vi "Read settings.vi"(8 "error in (no error)":errorcluster, 9 "force loading?":bool=TRUE, 10 "settings name":string, 11 "Autofocus in":refnum<class "Autofocus.lvclass">) -> (0 "error out":errorcluster, 1 "loaded?":bool, 2 "setting name":string, 3 "Autofocus out":refnum<class "Autofocus.lvclass">)   [LabVIEW 2012, in "Autofocus.lvclass"]
uses:
  Autofocus.lvclass
  <vilib>/Distrio/Murmex/Murmex/Murmex.lvclass
  Autofocus.lvclass/Autofocus.ctl
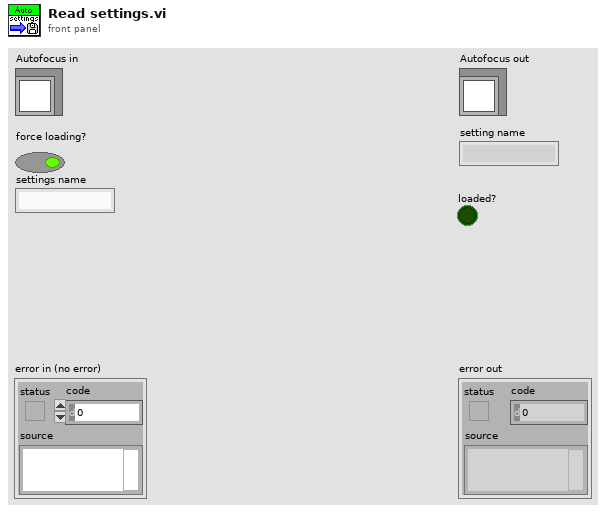
[diagram p1: front panel]
types:
  T1 = typedef "Autofocus.lvclass/settings cluster.ctl" = cluster{"Sharpness measure":T2, "ROI size":T3, "Search Algorithm":T4, "Region sampling":bool, "HC step size":dbl[unit], "current_position_focus":dbl[unit], "threshold":dbl, "brightest percentage":dbl, "number_of_checkpoints":u16, "current_stack_x":dbl[unit], "current_stack_y":dbl[unit], "curent_stack_z1":dbl[unit], "current_stack_z2":dbl[unit], "number_of_stacks":u16, "focus_start":dbl[unit], "focus_stop":dbl[unit], "frames_focus_stack":u16, "Image acquisition mode":T5, "frame rate":dbl[unit]}
  T2 = typedef "Autofocus.lvclass/Sharpness Measure.ctl" = enum16{"Vol4", "Gradient Square"}
  T3 = typedef "Autofocus.lvclass/ROI size.ctl" = u16
  T4 = typedef "Autofocus.lvclass/Search algorithm.ctl" = enum16{"Hill Climbing", "HC+GS"}
  T5 = typedef "Autofocus.lvclass/image acquisition mode.ctl" = enum16{"Focus Stack", "Single Frame"}
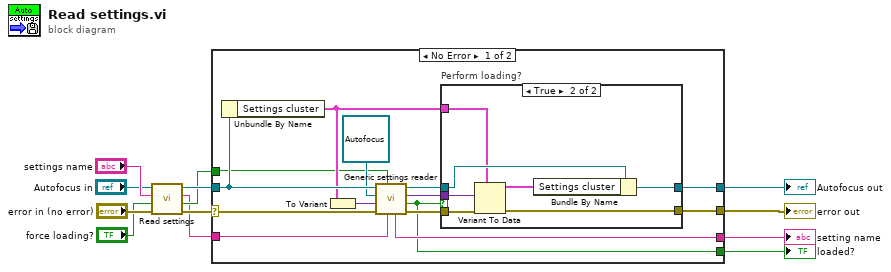
[diagram p0: block diagram]
diagram:
  n1 = call-parent "Read settings.vi"("error in (no error)"="error in (no error)", "force loading?"="force loading?", "settings name"="settings name", "Murmex in"="Autofocus in") -> ("error out"=w9:errorcluster, "loaded?"=w4:bool, "setting name"=w3:string, "Murmex out"=w8:refnum<class "Autofocus.lvclass">)  [unwired: 4 in]
  n2 = case shown="No Error" w9 {
    selector: w9 -> [w26 w37]
    tunnel: w8 -> [w25 w36]
    tunnel: [w18 w37] -> w7
    tunnel: [w17 w36] -> w6
    tunnel: w4 -> [w14 _]
    tunnel: w3 -> [w16 _]
    tunnel: [w15 _] -> w2
    tunnel: [w13 _] -> w1
    frame No Error {
      n3 = Unbundle By Name(w25) -> ("Settings cluster"=w19:T1)
      n4 = To Variant(anything=w19) -> (Variant=w24:variant)
      n5 = call <vilib>:"Generic settings reader.vi"("settings name"=w16, "force loading?"=w14, "error in (no error)"=w26, "settings cluster variant"=w24, "inheritance level"=refnum<class "Autofocus.lvclass"> refnum ("Autofocus.lvclass"), "Murmex in"=w25) -> ("error out"=w22:errorcluster, "loaded?"=w13:bool, "settings data (variant)"=w21:variant, "Murmex out"=w20:refnum<class "Autofocus.lvclass">, "setting name"=w15:string)  [unwired: 1 in]
      n6 = case "Perform loading?" shown="True" w13 {
        tunnel: [w28 w34] -> w18
        tunnel: [w27 w33] -> w17
        tunnel: w22 -> [w28 w30]
        tunnel: w20 -> [w27 w32]
        tunnel: w21 -> [_ w31]
        tunnel: w19 -> [_ w29]
        frame False {
        }
        frame True {
          n7 = Variant To Data(error in=w30, type=w29, Variant=w31) -> (data=w35:T1, error out=w34:errorcluster)
          n8 = Bundle By Name(cluster=w32, "Settings cluster"=w35) -> (w33:refnum<class "Autofocus.lvclass">)
        }
      }
    }
    frame Error {
    }
  }
  "error out" <- w7
  "Autofocus out" <- w6
  "setting name" <- w2
  "loaded?" <- w1
